vi "Start.vi"(8 "error in":errorcluster, 9 "timeout (-1)":i32=-1, 11 "Standard Engine in":refnum<class "synchronous engine runtime.lvclass">) -> (0 "error out":errorcluster, 3 "Standard Engine out":refnum<class "synchronous engine runtime.lvclass">)   [LabVIEW 2013, in "synchronous engine runtime.lvclass"]
uses:
  synchronous engine runtime.lvclass
  Commands.ctl
  notifier.ctl
  Engine Runtime/Execution States.ctl
  synchronous engine runtime.lvclass/synchronous engine runtime.ctl
  Standard Engine.vi
  Engine Runtime/Engine Runtime Interface.lvclass
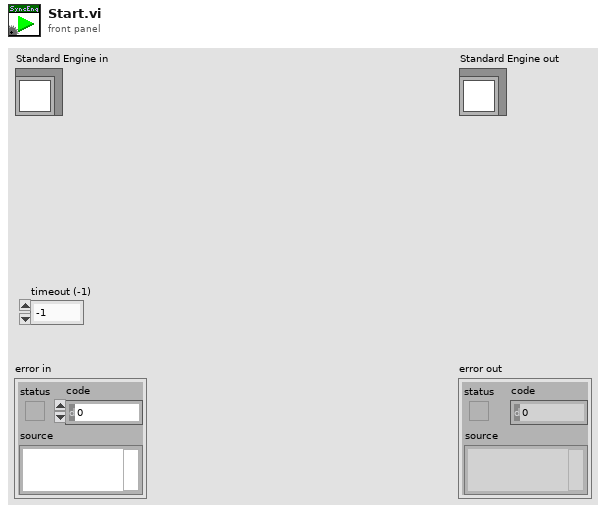
[diagram p1: front panel]
types:
  T1 = typedef "synchronous engine runtime.lvclass/notifier.ctl" = cluster{"Engine State":T2, "error constant":errorcluster}
  T2 = typedef "Engine Runtime Interface.lvclass/Execution States.ctl" = enum16{"Initializing", "Paused (Initialized)", "Running", "Set Safe Outputs", "Uninitializing", "Stopped (Uninitialized)", "Error (Uninitialized)", "Safe State (Uninitialized)", "Closed"}
  T3 = typedef "synchronous engine runtime.lvclass/Commands.ctl" = enum16{"Start", "Pause", "Safe State", "Normal", "Stop", "Shutdown"}
  T4 = typedef "synchronous engine runtime.lvclass/Engine Data.ctl" = cluster{"Main Tag Data":T5, "Module Info":T6, "Safe State?":bool, "engine timing source":refnum<class "TBM timing source.lvclass">, "Processor":i32, "Priority":i32, "dT":u32}
  T5 = typedef "tag bus.lvlib/data table.lvlib/data table.ctl" = cluster{"Double":dbl[], "Single":sgl[], "I64":i64[], "I32":i32[], "I16":i16[], "I8":i8[], "U64":u64[], "U32":u32[], "U16":u16[], "U8":u8[], "Boolean":bool[], "String":string[], "Array of Double":cluster{"DBL Array":dbl[]}[], "Array of Single":cluster{"SGL Array":sgl[]}[], "Array of I64":cluster{"I64 Array":i64[]}[], "Array of I32":cluster{"I32 Array":i32[]}[], "Array of I16":cluster{"I16 Array":i16[]}[], "Array of I8":cluster{"I8 Array":i8[]}[], "Array of U64":cluster{"U64 Array":u64[]}[], "Array of U32":cluster{"U32 Array":u32[]}[], "Array of U16":cluster{"U16 Array":u16[]}[], "Array of U8":cluster{"U8 Array":u8[]}[], "Array of Boolean":cluster{"Boolean Array":bool[]}[], "Array of String":cluster{"String Array":string[]}[]}
  T6 = typedef "synchronous engine runtime.lvclass/Module Execution Info.ctl" = cluster{"Tag Bus Modules":refnum<class "TBM module execution interface.lvclass">[], "Input Method Indices":i32[], "Process Method Indices":i32[], "Output Method Indices":i32[], "Input Transfer Specifications":T7[], "Parameter Transfer Specifications":T7[], "Result Transfer Specifications":T7[], "Output Transfer Specifications":T7[], "Module Errors":errorcluster[], "UID":string}
  T7 = typedef "synchronous engine runtime.lvclass/Data Table with Transfer Spec.ctl" = cluster{"Data Table":T5, "Transfer Specification":T8[]}
  T8 = typedef "tag bus.lvlib/data table.lvlib/transfer specification.ctl" = cluster{"data type":T9, "sink indices":i32[], "source indices":i32[]}
  T9 = typedef "tag bus.lvlib/tag descriptor.lvclass/Data Type.ctl" = enum16{"Double", "Single", "I64", "I32", "I16", "I8", "U64", "U32", "U16", "U8", "Boolean", "String", "Array of Double", "Array of Single", "Array of I64", "Array of I32", "Array of I16", "Array of I8", "Array of U64", "Array of U32", "Array of U16", "Array of U8", "Array of Boolean", "Array of String"}
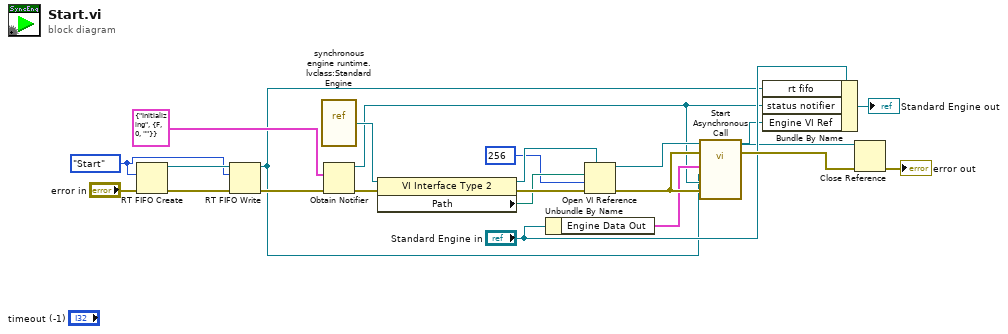
[diagram p0: block diagram]
diagram:
  w1 = Commands."Start" ("element")
  n1 = RT FIFO Create(1:w1, 3:"error in") -> (8:w3:refnum<k33>, 11:w15:errorcluster)  [unwired: 6 in, 1 out]
  n2 = RT FIFO Write(0:w3, 1:w1, 3:w15) -> (8:w2:refnum<k33>, 11:w4:errorcluster)  [unwired: 2 in, 2 out]
  n3 = vi-ref "synchronous engine runtime.lvclass:Standard Engine.vi"() -> (w22:refnum<vi>)
  n4 = Obtain Notifier(notification data type=T1 {"Engine State"=enum."Initializing", "error constant"={"status"=FALSE, "code"=0, "source"=""}}, error in (no error)=w4) -> (notifier out=w7:refnum<notifier>, error out=w9:errorcluster)  [unwired: 2 in, 1 out]
  n5 = property class="VI Interface Type 2"(reference=w22, error in=w9) -> (reference out=w18:refnum<vi>, error out=w20:errorcluster, "Path"=w19:path)
  n6 = Unbundle By Name("Standard Engine in") -> ("Engine Data Out"=w10:T4)
  n7 = Open VI Reference(type specifier VI Refnum (for type only)=w18, vi path=w19, options=256, error in (no error)=w20) -> (vi reference=w14:refnum<vi>, error out=w12:errorcluster)  [unwired: 2 in]
  n8 = call-by-ref "Start Asynchronous Call"(reference=w14, error in=w12, "error in"=w12, "status notifier"=w7, "rt fifo"=w2, "Engine Data"=w10) -> (reference out=w5:refnum<vi>, error out=w16:errorcluster)  [unwired: 7 in, 1 out]
  n9 = Bundle By Name(cluster="Standard Engine in", "rt fifo"=w2, "status notifier"=w7, "Engine VI Ref"=w5) -> (→"Standard Engine out":refnum<class "synchronous engine runtime.lvclass">)
  n10 = Close Reference(reference=w5, error in (no error)=w16) -> (error out=→"error out":errorcluster)
